vi "Execute.vi"(6 "Error":errorcluster, 7 "Message":refnum<class "Message.lvclass">, 11 "Actor":refnum<class "Actor.lvclass">) -> (3 "Actor":refnum<class "Actor.lvclass">, 4 "Error":errorcluster, 5 "Message":refnum<class "Message.lvclass">)   [LabVIEW 2020, in "_Template.lvlib" / "{{Message}}.lvlib" / "Message.lvclass"]
uses:
  Message.lvclass
  jettl/jettl/Actor/Actor.lvclass
  ActorMessage/ActorMessage.lvclass
  Message.lvclass/Message.ctl
panel:
  # "This front panel should not be manipulated."
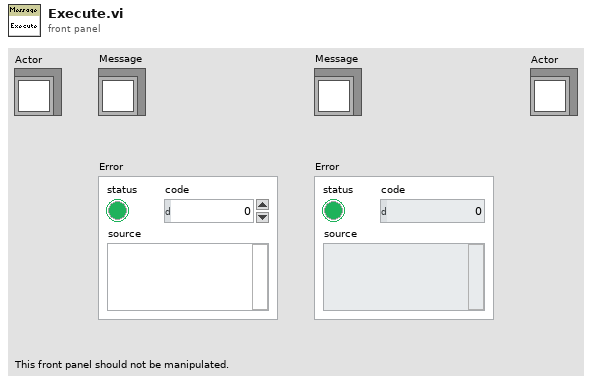
[diagram p1: front panel]
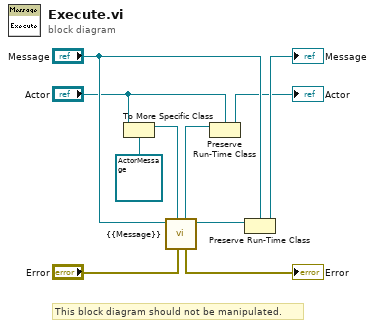
[diagram p0: block diagram]
diagram:
  # "This block diagram should not be manipulated."
  n1 = To More Specific Class(target class=refnum<class "ActorMessage.lvclass"> refnum ("_Template.lvlib:Templates.lvlib:TEMPLATE jettl Msg.lvlib:TEMPLATE jettl Msg.lvclass"), reference="Actor") -> (specific class reference=w7:refnum<class "ActorMessage.lvclass">)  [unwired: 1 in, 1 out]
  n2 = call-dynamic "{{Message}}.vi"("Error"="Error", "ActorMessage"=w7, "Message"="Message") -> ("Message"=w4:refnum<class "Message.lvclass">, "Error"=→"Error":errorcluster, "ActorMessage"=w6:refnum<class "ActorMessage.lvclass">)  [unwired: 6 in]
  n3 = Preserve Run-Time Class(object in=w6, 2:"Actor") -> (object out=→"Actor":refnum<class "Actor.lvclass">)  [unwired: 1 in, 1 out]
  n4 = Preserve Run-Time Class(object in=w4, 2:"Message") -> (object out=→"Message":refnum<class "Message.lvclass">)  [unwired: 1 in, 1 out]
